vi "spin_diode_effect.vi"() -> ()   [LabVIEW 2017]
doc: "Use this template to build a simple state machine design pattern. Each state executes code and determines which state to transition to."
uses:
  <userlib>/niRF/niQuickSyn/Core/Properties/VISA Handle/PropertyType.ctl
  <userlib>/niRF/niQuickSyn/Core/Properties/VISA Handle/VISA Handle.lvclass
  controls/Instruments.ctl
  controls/State.ctl
  <userlib>/niRF/niQuickSyn/QuickSyn API.lvlib
  <userlib>/niRF/niQuickSyn/Core/QuickSyn.lvclass
  <userlib>/niRF/niQuickSyn/Core/Typedefs/Session Handle.ctl
  <vilib>/DAQmx/create/channels.llb/DAQmx Create Channel (AO-Voltage-Basic).vi
  <vilib>/DAQmx/configure/timing.llb/DAQmx Timing (Sample Clock).vi
  <vilib>/DAQmx/create/channels.llb/DAQmx Create Channel (AI-Voltage-Basic).vi
  <vilib>/DAQmx/configure/trigger.llb/DAQmx Start Trigger (None).vi
  <userlib>/niRF/niQuickSyn/Core/Properties/AM State/PropertyType.ctl
  <userlib>/niRF/niQuickSyn/Core/Properties/AM State/AM State.lvclass
  <userlib>/niRF/niQuickSyn/Core/Properties/FM Sensitivity/PropertyType.ctl
  <userlib>/niRF/niQuickSyn/Core/Properties/FM Sensitivity/FM Sensitivity.lvclass
  <vilib>/measure/NI_MABase.lvlib
  <vilib>/DAQmx/write.llb/DAQmx Write (Analog Wfm 1Chan NSamp).vi
  <userlib>/niRF/niQuickSyn/Core/Properties/RF Output/PropertyType.ctl
  <userlib>/niRF/niQuickSyn/Core/Properties/RF Output/RF Output.lvclass
panel:
  out "Type of magnet":bool
  in  "Field, Oe":dbl=13.0 caption="Stop H Field (Oe)" min=-10.0 max=13.0 step=0.5 format="%#_6f"
  in  "Generator Session":T1
  in  "error in (no error)":errorcluster
  out "Status":string="Shutting down..."
  in  "Exit Button":bool
  in  "Save Button":bool
  in  "Start Button":bool
  in  "Stop Button":bool
  in  "Generator Power, dBm":dbl=13.0 caption="Stop H Field (Oe)" min=-10.0 max=13.0 step=0.5 format="%#_6f"
  in  "Modulation Amplitude, V":dbl=10.0 caption="Stop H Field (Oe)" min=0.0 max=10.0 format="%#_6f"
  in  "Generator Frequency, GHz":dbl=20.0 caption="Stop H Field (Oe)" min=0.5 max=20.0 format="%#_6f"
  in  "Modulation Frequency, KHz":dbl min=0.0 max=0.0 format="%#_6f"
  in  "Switch port":refnum<visa-resource-name>="COM6"
  in  "AKIP":refnum<visa-resource-name>="AKIP"
  in  "DAQ channel AI":tag="DAQ6363/ai4"
  in  "DAQ channel AO":tag="DAQ6363/ao0"
  in  "DAQ AI task":refnum<k21>
  in  "DAQ AO task":refnum<k21>
  in  "Genarator name":T2="QuickSyn_generator"
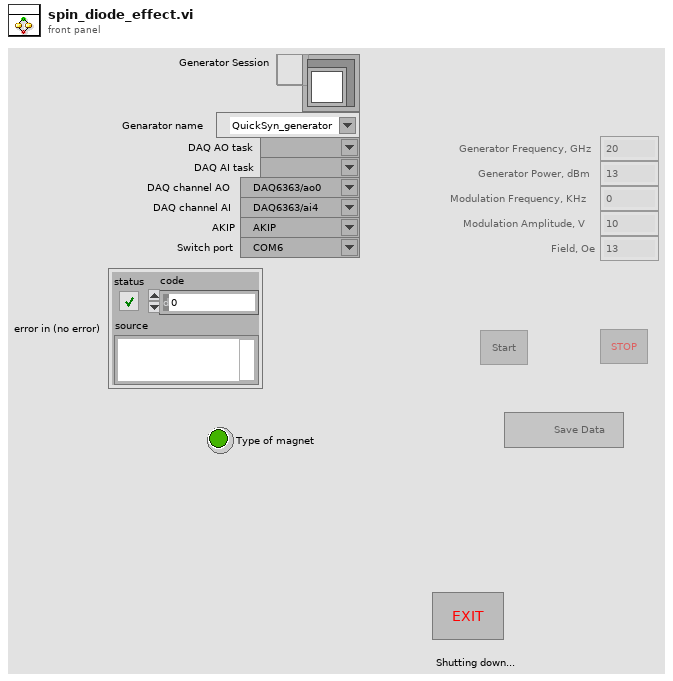
[diagram p1: front panel]
types:
  T1 = typedef "QuickSyn API.lvlib/QuickSyn.lvclass/Session Handle.ctl" = refnum<data-value>
  T2 = typedef "QuickSyn API.lvlib/VISA Handle.lvclass/PropertyType.ctl" = refnum<visa-resource-name>
  T3 = typedef "State.ctl" = enum16{"Init", "Idle", "Starting", "Measure", "Stopping", "Shutdown"}
  T4 = typedef "Instruments.ctl" = cluster{"Genarator name":T2, "DAQ AO task":refnum<k21>, "DAQ AI task ":refnum<k21>, "DAQ channel AO ":tag, "DAQ channel AI":tag, "AKIP":refnum<visa-resource-name>, "Switch port":refnum<visa-resource-name>, "Generator Session":T1}
  T5 = typedef "QuickSyn API.lvlib/FM Sensitivity.lvclass/PropertyType.ctl" = dbl
  T6 = typedef "QuickSyn API.lvlib/AM State.lvclass/PropertyType.ctl" = enum16{"Disabled", "Enabled"}
  T7 = enum16{"Sine Wave", "Triangle Wave", "Square Wave", "Sawtooth Wave"}
  T8 = typedef "QuickSyn API.lvlib/RF Output.lvclass/PropertyType.ctl" = bool
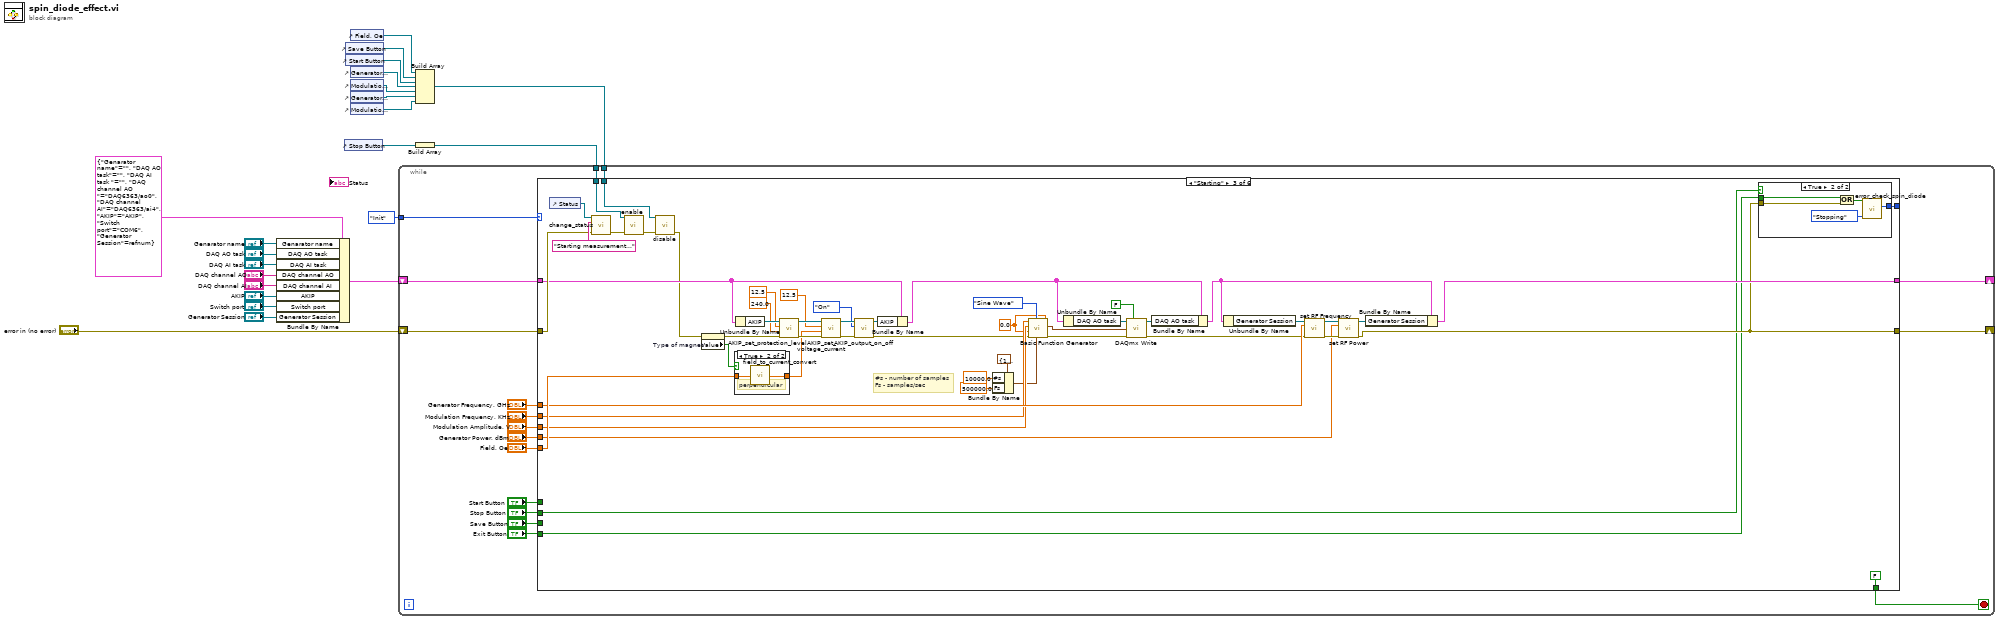
[diagram p0: block diagram]
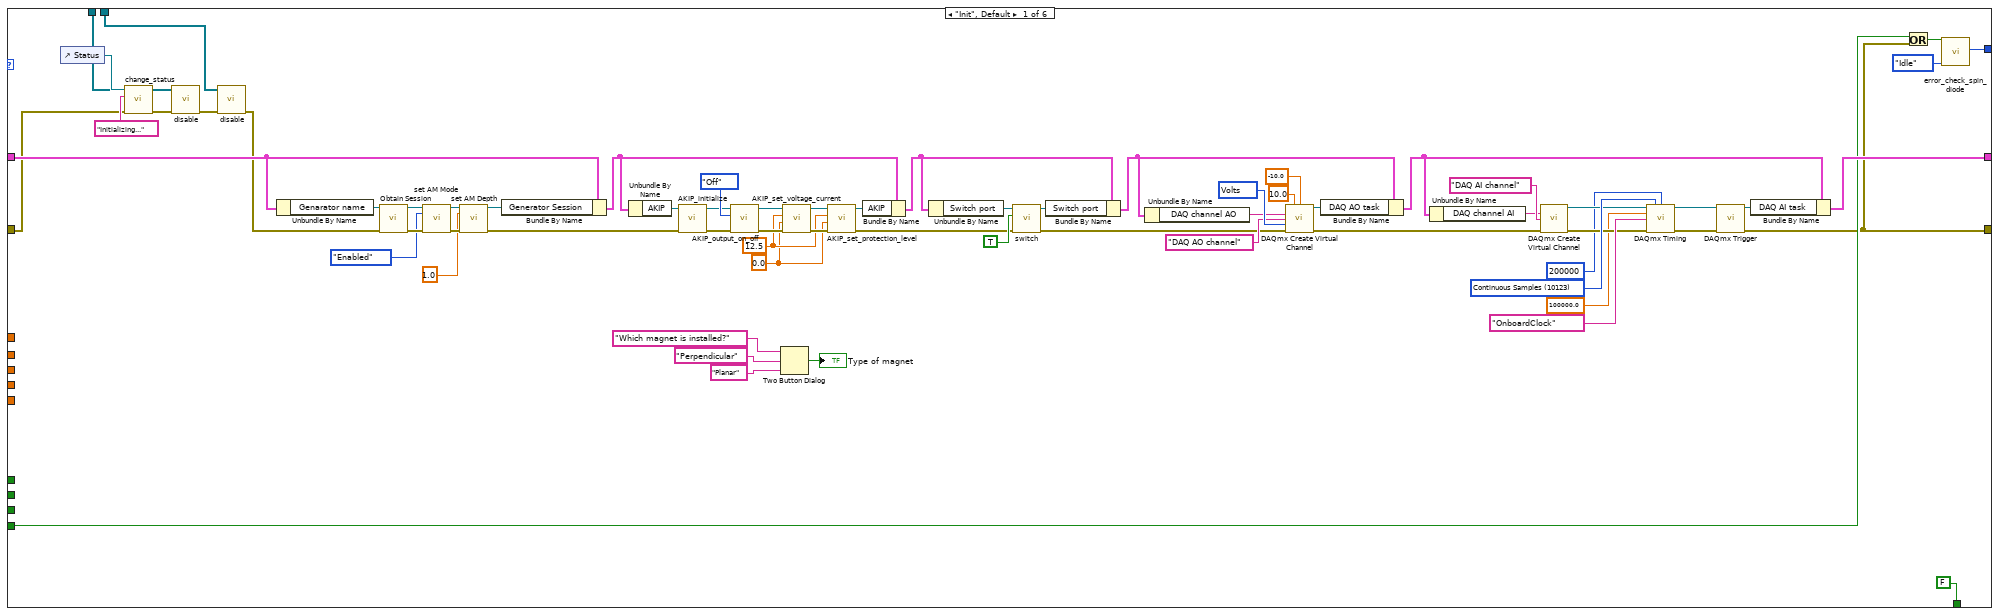
[diagram p2: hidden frame]
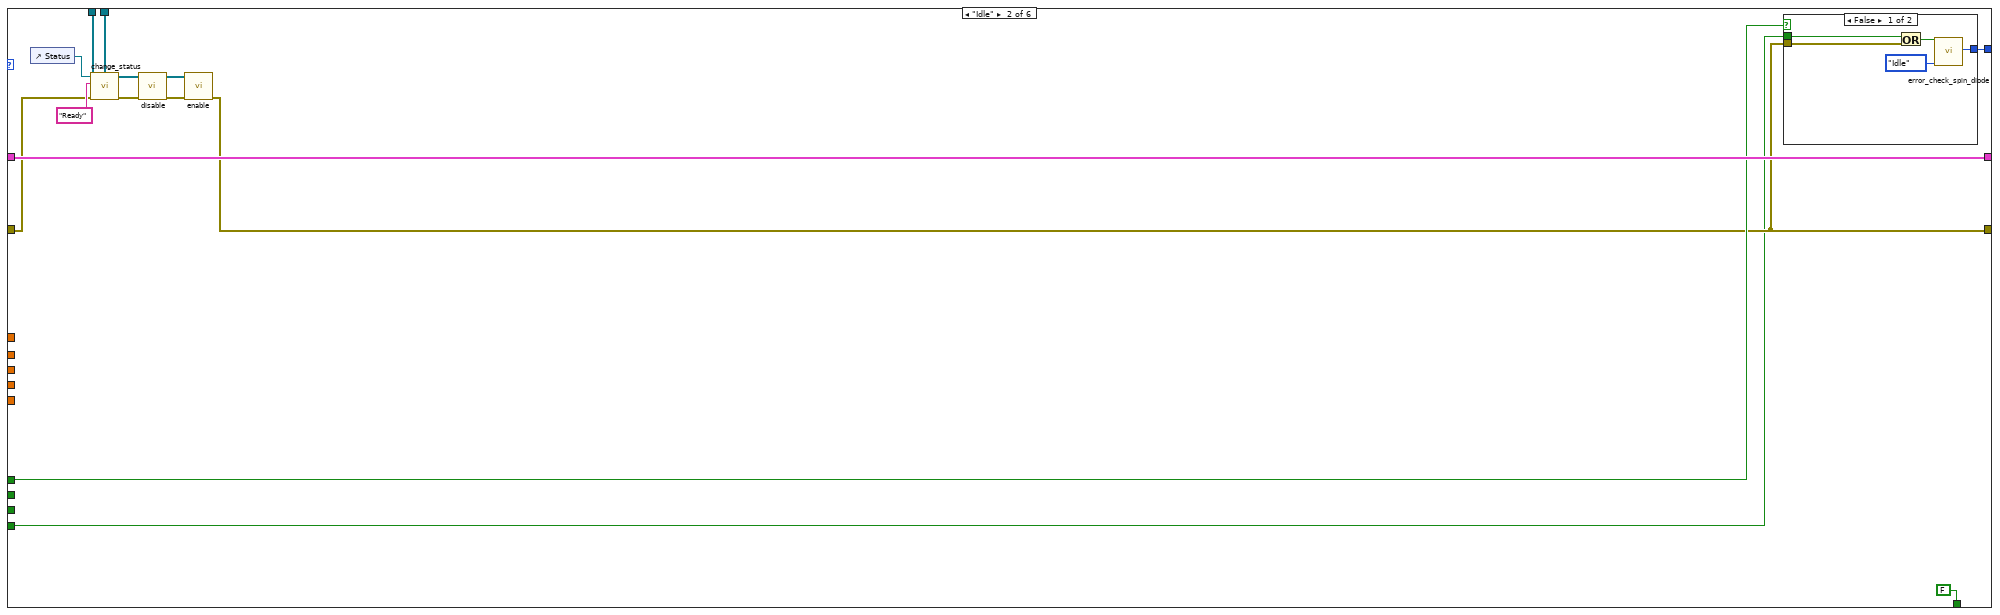
[diagram p3: hidden frame]
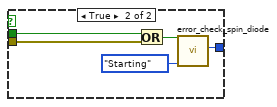
[diagram p4: hidden frame]
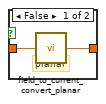
[diagram p5: hidden frame]
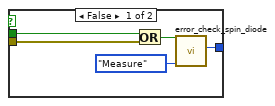
[diagram p6: hidden frame]
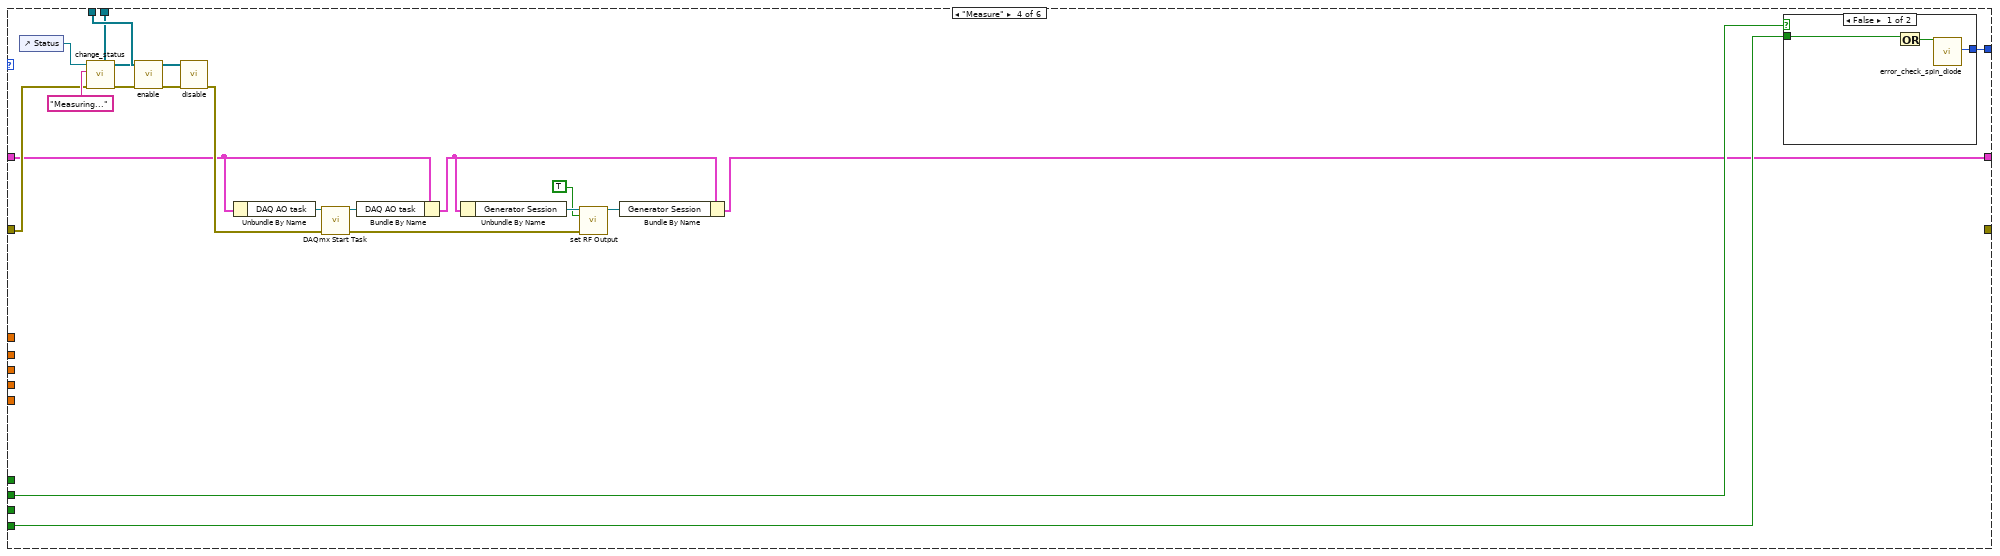
[diagram p7: hidden frame]
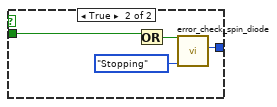
[diagram p8: hidden frame]
diagram:
  n1 = Bundle By Name(cluster=T4 {"Genarator name"="", "DAQ AO task"="", "DAQ AI task "="", "DAQ channel AO "="DAQ6363/ao0", "DAQ channel AI"="DAQ6363/ai4", "AKIP"="AKIP", "Switch port"="COM6", "Generator Session"=refnum}, "Genarator name"="Genarator name", "DAQ AO task"="DAQ AO task", "DAQ AI task"="DAQ AI task", "DAQ channel AO"="DAQ channel AO", "DAQ channel AI"="DAQ channel AI", "AKIP"="AKIP", "Switch port"="Switch port", "Generator Session"="Generator Session") -> (w14:T4)
  n2 = control-ref of="Stop Button"() -> (w3:refnum<vi>)
  n3 = control-ref of="Save Button"() -> (w12:refnum<vi>)
  n4 = control-ref of="Start Button"() -> (w2:refnum<vi>)
  n5 = control-ref of="Field, Oe"() -> (w1:refnum<vi>)
  n6 = control-ref of="Generator Power, dBm"() -> (w11:refnum<vi>)
  n7 = control-ref of="Modulation Amplitude, V"() -> (w10:refnum<vi>)
  n8 = control-ref of="Generator Frequency, GHz"() -> (w9:refnum<vi>)
  n9 = control-ref of="Modulation Frequency, KHz"() -> (w8:refnum<vi>)
  n10 = Build Array(w1, w12, w2, w11, w10, w9, w8) -> (w6:refnum<vi>[])
  n11 = Build Array(w3) -> (w7:refnum<vi>[])
  n12 = while {
    tunnel: State."Init" -> [w38]
    tunnel: w7 -> [w29]
    tunnel: w6 -> [w28]
    shift-right: [w27] -> _
    shift-left: "error in (no error)" -> [w26]
    shift-right: [w23] -> _
    shift-left: w14 -> [w39]
    stop <- w25 stop-if-true
    n13 = case shown="\"Starting\"" w38 {
      tunnel: w39 -> [w96 w119 w163 w202 w223 w224]
      tunnel: [w56 w119 w152 w198 w223 w224] -> w23
      tunnel: [w106 w109 w181 w208 _ _] -> _
      tunnel: "Generator Frequency, GHz" -> [_ _ w154 _ _ _]
      tunnel: "Modulation Frequency, KHz" -> [_ _ w150 _ _ _]
      tunnel: "Modulation Amplitude, V" -> [_ _ w149 _ _ _]
      tunnel: "Generator Power, dBm" -> [_ _ w153 _ _ _]
      tunnel: "Start Button" -> [_ w110 _ _ _ _]
      tunnel: "Stop Button" -> [_ _ w132 w207 _ _]
      tunnel: "Save Button" -> [_ _ _ _ _ _]
      tunnel: "Exit Button" -> [w55 w107 w133 w206 _ _]
      tunnel: w29 -> [w99 w113 w175 w211 _ _]
      tunnel: w28 -> [w98 w112 w174 w210 _ _]
      tunnel: [w54 w108 w134 _ _ _] -> w27
      tunnel: w26 -> [w53 w114 w176 w209 _ _]
      tunnel: [FALSE FALSE FALSE _ _ _] -> w25
      tunnel: "Field, Oe" -> [_ _ w159 _ _ _]
      frame "Init", Default {
        w74 = 10123 items=["Finite Samples"=10178, "Continuous Samples"=10123, "Hardware Timed Single Point"=12522] ("sample mode")
        w75 = 10348 items=["Volts"=10348, "From Custom Scale"=10065] ("units")
        w87 = 0.0 ("Current")
        w88 = 12.5 ("Voltage")
        n14 = control-ref of="Status"() -> (w103:refnum<vi>)
        n15 = call "change_status.vi"("error in (no error)"=w53, "String"="Initializing...", "String in"=w103) -> ("error out"=w101:errorcluster)  [unwired: 8 in]
        n16 = call "disable.vi"("error in (no error)"=w101, "Array"=w99) -> ("error out"=w100:errorcluster)  [unwired: 9 in]
        n17 = call "disable.vi"("error in (no error)"=w100, "Array"=w98) -> ("error out"=w95:errorcluster)  [unwired: 9 in]
        n18 = Unbundle By Name(w96) -> ("Genarator name"=w97:T2)
        n19 = call <userlib>:"Obtain Session.vi"("VISA resource name"=w97, "error in (no error)"=w95) -> ("Session Handle"=w47:T1, "error out"=w46:errorcluster)  [unwired: 12 in]
        n20 = call <userlib>:"set AM Mode.vi"("Session Handle in"=w47, "AM State"=PropertyType."Enabled", "error in (no error)"=w46) -> ("Session Handle out"=w44:T1, "error out"=w43:errorcluster)  [unwired: 11 in]
        n21 = call <userlib>:"set AM Depth.vi"("Session Handle in"=w44, "AM Depth"=T5 1.0, "error in (no error)"=w43) -> ("Session Handle out"=w42:T1, "error out"=w41:errorcluster)  [unwired: 11 in]
        n22 = Bundle By Name(cluster=w96, "Generator Session"=w42) -> (w83:T4)
        n23 = Unbundle By Name(w83) -> ("AKIP"=w94:refnum<visa-resource-name>)
        n24 = call "AKIP_initialize.vi"("error in (no error)"=w41, "VISA Refnum in"=w94) -> ("error out"=w85:errorcluster, "VISA Refnum out"=w86:refnum<visa-resource-name>)  [unwired: 8 in]
        n25 = call "AKIP_output_on_off.vi"("error in (no error)"=w85, "Enum"=enum16{"On", "Off"}."Off", "VISA Refnum in"=w86) -> ("error out"=w91:errorcluster, "VISA Refnum out"=w92:refnum<visa-resource-name>)  [unwired: 7 in]
        n26 = Two Button Dialog(message="Which magnet is installed?", 1:"Planar" ("F button name (\"Cancel\")"), 2:"Perpendicular" ("T button name (\"OK\")")) -> (T button?=→"Type of magnet":bool)
        n27 = call "AKIP_set_voltage_current.vi"("error in (no error)"=w91, "Current"=w87, "Voltage"=w88, "VISA resource name (in)"=w92) -> ("error out"=w90:errorcluster, "VISA resource name (out)"=w89:refnum<visa-resource-name>)  [unwired: 6 in]
        n28 = call "AKIP_set_protection_level.vi"("error in (no error)"=w90, "Current Protection Level"=w87, "Voltage Protection Level"=w88, "VISA resource name (in)"=w89) -> ("error out"=w79:errorcluster, "VISA resource name (out)"=w84:refnum<visa-resource-name>)  [unwired: 6 in]
        n29 = Bundle By Name(cluster=w83, "AKIP"=w84) -> (w78:T4)
        n30 = Unbundle By Name(w78) -> ("Switch port"=w81:refnum<visa-resource-name>)
        n31 = call "switch.vi"("error in (no error)"=w79, "Positive?"=TRUE, "Switch port (in)"=w81) -> ("error out"=w64:errorcluster, "Switch port (out)"=w80:refnum<visa-resource-name>)  [unwired: 7 in]
        n32 = Bundle By Name(cluster=w78, "Switch port"=w80) -> (w61:T4)
        n33 = Unbundle By Name(w61) -> ("DAQ channel AO"=w63:tag)
        n34 = call-poly <vilib>:"DAQmx Create Virtual Channel.vi"("maximum value"=10.0, "minimum value"=-10.0, "physical channels"=w63, "name to assign"="DAQ AO channel", "units"=w75, "error in"=w64) -> ("task out"=w62:refnum<k21>, "error out"=w60:errorcluster)  [unwired: 8 in]
        n35 = Bundle By Name(cluster=w61, "DAQ AO task"=w62) -> (w57:T4)
        n36 = Unbundle By Name(w57) -> ("DAQ channel AI"=w59:tag)
        n37 = call-poly <vilib>:"DAQmx Create Virtual Channel.vi"("physical channels"=w59, "name to assign"="DAQ AI channel", "error in"=w60) -> ("task out"=w72:refnum<k21>, "error out"=w71:errorcluster)  [unwired: 11 in]
        n38 = call-poly <vilib>:"DAQmx Timing.vi"("task/channels in"=w72, "sample mode"=w74, "samples per channel"=200000, "rate"=100000.0, "source"=tag "OnboardClock", "error in"=w71) -> ("task out"=w70:refnum<k21>, "error out"=w69:errorcluster)  [unwired: 8 in]
        n39 = call-poly <vilib>:"DAQmx Trigger.vi"("task/channels in"=w70, "error in"=w69) -> ("task out"=w58:refnum<k21>, "error out"=w54:errorcluster)  [unwired: 12 in]
        n40 = Bundle By Name(cluster=w57, "DAQ AI task"=w58) -> (w56:T4)
        n41 = Or(x=w55, y=w54) -> (x .or. y?=w104:bool)
        n42 = call "error_check_spin_diode.vi"("State"=State."Idle", "Boolean"=w104) -> ("Result state"=w106:T3)  [unwired: 9 in]
      }
      frame "Idle" {
        n43 = control-ref of="Status"() -> (w115:refnum<vi>)
        n44 = call "change_status.vi"("error in (no error)"=w114, "String"="Ready", "String in"=w115) -> ("error out"=w117:errorcluster)  [unwired: 8 in]
        n45 = call "disable.vi"("error in (no error)"=w117, "Array"=w113) -> ("error out"=w116:errorcluster)  [unwired: 9 in]
        n46 = call "enable.vi"("error in (no error)"=w116, "Array"=w112) -> ("error out"=w108:errorcluster)  [unwired: 9 in]
        n47 = case shown="False" w110 {
          tunnel: [w122 w127] -> w109
          tunnel: w108 -> [w121 w126]
          tunnel: w107 -> [w120 w125]
          frame False {
            n48 = Or(x=w120, y=w121) -> (x .or. y?=w123:bool)
            n49 = call "error_check_spin_diode.vi"("State"=State."Idle", "Boolean"=w123) -> ("Result state"=w122:T3)  [unwired: 9 in]
          }
          frame True {
            n50 = Or(x=w125, y=w126) -> (x .or. y?=w128:bool)
            n51 = call "error_check_spin_diode.vi"("State"=State."Starting", "Boolean"=w128) -> ("Result state"=w127:T3)  [unwired: 9 in]
          }
        }
      }
      frame "Starting" {
        w130 = 0.0 ("phase")
        # "#s - number of samples\nFs - samples/sec"
        n52 = control-ref of="Status"() -> (w177:refnum<vi>)
        n53 = call "change_status.vi"("error in (no error)"=w176, "String"="Starting measurement...", "String in"=w177) -> ("error out"=w179:errorcluster)  [unwired: 8 in]
        n54 = call "enable.vi"("error in (no error)"=w179, "Array"=w175) -> ("error out"=w178:errorcluster)  [unwired: 9 in]
        n55 = call "disable.vi"("error in (no error)"=w178, "Array"=w174) -> ("error out"=w162:errorcluster)  [unwired: 9 in]
        n56 = property on="Type of magnet" class="Bool (strict)"(error in=w162) -> (error out=w161:errorcluster, "Value"=w160:bool)  [unwired: 1 in, 1 out]
        n57 = case shown="True" w160 {
          tunnel: [w183 w185] -> w158
          tunnel: w159 -> [w182 w184]
          frame False {
            # "planar"
            n58 = call "field_to_current_convert_planar.vi"("Field, Oe"=w182) -> ("Current, A"=w183:dbl)
          }
          frame True {
            # "perpendicular"
            n59 = call "field_to_current_convert.vi"("Field, Oe"=w184) -> ("Current, A"=w185:dbl)
          }
        }
        n60 = Unbundle By Name(w163) -> ("AKIP"=w173:refnum<visa-resource-name>)
        n61 = call "AKIP_set_protection_level.vi"("error in (no error)"=w161, "Current Protection Level"=240.0 ("Voltage Protection Level"), "Voltage Protection Level"=12.5 ("Current Protection Level"), "VISA resource name (in)"=w173) -> ("error out"=w171:errorcluster, "VISA resource name (out)"=w172:refnum<visa-resource-name>)  [unwired: 6 in]
        n62 = call "AKIP_set_voltage_current.vi"("error in (no error)"=w171, "Current"=w158, "Voltage"=12.5, "VISA resource name (in)"=w172) -> ("error out"=w168:errorcluster, "VISA resource name (out)"=w169:refnum<visa-resource-name>)  [unwired: 6 in]
        n63 = call "AKIP_output_on_off.vi"("error in (no error)"=w168, "Enum"=enum16{"On", "Off"}."On", "VISA Refnum in"=w169) -> ("error out"=w144:errorcluster, "VISA Refnum out"=w164:refnum<visa-resource-name>)  [unwired: 7 in]
        n64 = Bundle By Name(cluster=w163, "AKIP"=w164) -> (w139:T4)
        n65 = Bundle By Name(cluster=cluster{"Fs":dbl, "#s":dbl} {"Fs"=1000.0, "#s"=1000.0} ("sampling info"), "#s"=10000.0, "Fs"=500000.0) -> (w145:cluster{"Fs":dbl, "#s":dbl})
        n66 = call <vilib>:"Basic Function Generator.vi"("offset"=w130, "sampling info"=w145, "signal type"=T7."Sine Wave", "error in (no error)"=w144, "phase"=w130, "amplitude"=w149, "frequency"=w150) -> ("error out"=w142:errorcluster, "signal out"=w143:waveform(dbl))  [unwired: 2 in, 1 out]
        n67 = Unbundle By Name(w139) -> ("DAQ AO task"=w141:refnum<k21>)
        n68 = call-poly <vilib>:"DAQmx Write.vi"("task/channels in"=w141, "auto start"=FALSE, "data"=w143, "error in"=w142) -> ("task out"=w140:refnum<k21>, "error out"=w136:errorcluster)  [unwired: 9 in, 1 out]
        n69 = Bundle By Name(cluster=w139, "DAQ AO task"=w140) -> (w138:T4)
        n70 = Unbundle By Name(w138) -> ("Generator Session"=w157:T1)
        n71 = call <userlib>:"set RF Frequency.vi"("Session Handle in"=w157, "RF Frequency, Hz (200M)"=w154, "error in (no error)"=w136) -> ("Session Handle out"=w156:T1, "error out"=w155:errorcluster)  [unwired: 11 in]
        n72 = call <userlib>:"set RF Power.vi"("Session Handle in"=w156, "RF Power, dB (0)"=w153, "error in (no error)"=w155) -> ("Session Handle out"=w137:T1, "error out"=w134:errorcluster)  [unwired: 11 in]
        n73 = Bundle By Name(cluster=w138, "Generator Session"=w137) -> (w152:T4)
        n74 = case shown="True" w132 {
          tunnel: [w188 w193] -> w181
          tunnel: w133 -> [w187 w192]
          tunnel: w134 -> [w186 w191]
          frame False {
            n75 = Or(x=w187, y=w186) -> (x .or. y?=w189:bool)
            n76 = call "error_check_spin_diode.vi"("State"=State."Measure", "Boolean"=w189) -> ("Result state"=w188:T3)  [unwired: 9 in]
          }
          frame True {
            n77 = Or(x=w192, y=w191) -> (x .or. y?=w194:bool)
            n78 = call "error_check_spin_diode.vi"("State"=State."Stopping", "Boolean"=w194) -> ("Result state"=w193:T3)  [unwired: 9 in]
          }
        }
      }
      frame "Measure" {
        n79 = control-ref of="Status"() -> (w212:refnum<vi>)
        n80 = call "change_status.vi"("error in (no error)"=w209, "String"="Measuring...", "String in"=w212) -> ("error out"=w215:errorcluster)  [unwired: 8 in]
        n81 = call "enable.vi"("error in (no error)"=w215, "Array"=w211) -> ("error out"=w214:errorcluster)  [unwired: 9 in]
        n82 = call "disable.vi"("error in (no error)"=w214, "Array"=w210) -> ("error out"=w204:errorcluster)  [unwired: 9 in]
        n83 = Unbundle By Name(w202) -> ("DAQ AO task"=w205:refnum<k21>)
        n84 = call <vilib>:"DAQmx Start Task.vi"("task/channels in"=w205, "error in"=w204) -> ("task out"=w203:refnum<k21>, "error out"=w197:errorcluster)  [unwired: 12 in]
        n85 = Bundle By Name(cluster=w202, "DAQ AO task"=w203) -> (w199:T4)
        n86 = Unbundle By Name(w199) -> ("Generator Session"=w201:T1)
        n87 = call <userlib>:"set RF Output.vi"("Session Handle in"=w201, "RF Output (False)"=T8 TRUE, "error in (no error)"=w197) -> ("Session Handle out"=w200:T1)  [unwired: 11 in, 1 out]
        n88 = Bundle By Name(cluster=w199, "Generator Session"=w200) -> (w198:T4)
        n89 = case shown="False" w207 {
          tunnel: [w217 w220] -> w208
          tunnel: w206 -> [w216 w219]
          frame False {
            n90 = Or(x=w216) -> (x .or. y?=w218:bool)  [unwired: 1 in]
            n91 = call "error_check_spin_diode.vi"("Boolean"=w218) -> ("Result state"=w217:T3)  [unwired: 10 in]
          }
          frame True {
            n92 = Or(x=w219) -> (x .or. y?=w221:bool)  [unwired: 1 in]
            n93 = call "error_check_spin_diode.vi"("State"=State."Stopping", "Boolean"=w221) -> ("Result state"=w220:T3)  [unwired: 9 in]
          }
        }
      }
      frame "Stopping" {
      }
      frame "Shutdown" {
      }
    }
  }
